vi "Compile Asynchronous Execution Units.vi"(0 "Device Ref in":T2=18446744073709551615 format="%.0x", 1 "Asynchronous Execution Units":T3[](array[typedef]) {"Outgoing Channels" format="%.0x"; "Incoming Channels" format="%.0x"}, 3 "error in":errorcluster) -> (7 "Device Ref out":T2=18446744073709551615 format="%.0x", 8 "Compiled Asynchronous Execution Units":T1[](array[typedef]), 10 "error out":errorcluster)   [LabVIEW 2020, in "Communication Bus Template System Explorer.lvlib" / "Implementation.lvlib"]
uses:
  Implementation.lvlib
  <vilib>/NI VeriStand/Custom Device API/Custom Device Item Ref.ctl
  <vilib>/NI VeriStand/Custom Device API/Custom Device API.lvlib
  <vilib>/NI/NIVS Inline Async API/_Data Access System Explorer/Data Access System Explorer.lvlib
  Engine/Interfaces/Execution Unit/Execution Unit.lvclass
  Engine/Custom Device/Asynchronous Execution Unit Compiled Information.ctl
  Engine/Custom Device/Custom Device.lvlib
  Engine/Interfaces/Controls/Execution Unit Information.ctl
  Engine/Interfaces/Interfaces.lvlib
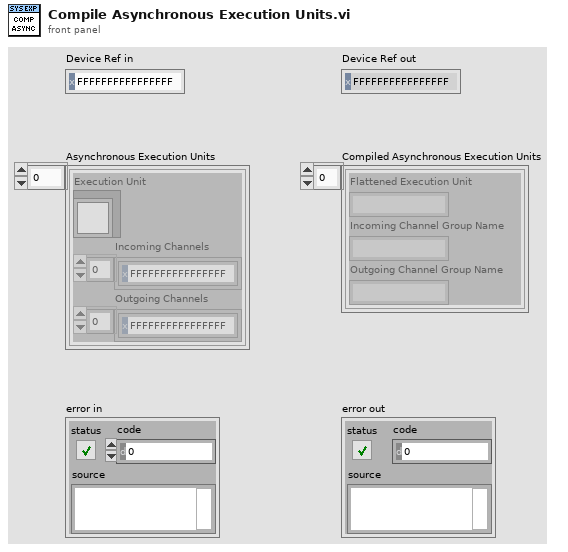
[diagram p1: front panel]
types:
  T1 = typedef "Communication Bus Template Engine.lvlib/Custom Device.lvlib/Asynchronous Execution Unit Compiled Information.ctl" = cluster{"Flattened Execution Unit":string, "Incoming Channel Group Name":string, "Outgoing Channel Group Name":string}
  T2 = typedef "Custom Device API.lvlib/Custom Device Item Ref.ctl" = u64
  T3 = typedef "Communication Bus Template Engine.lvlib/Interfaces.lvlib/Execution Unit Information.ctl" = cluster{"Execution Unit":refnum<class "Execution Unit.lvclass">, "Incoming Channels":T2[], "Outgoing Channels":T2[]}
  T4 = enum16{"Output/Write", "Input/Read", "Input/ReadWrite"}
  T5 = cluster{"Name":string, "Type":enum16{"Output/Write", "Input/Read", "Input/ReadWrite"}, "VS Refs":T2[]}
  T6 = cluster{"Name":string, "Type":enum16{"Output/Write", "Input/Read", "Input/ReadWrite"}, "VS Refs":T2[]}[]
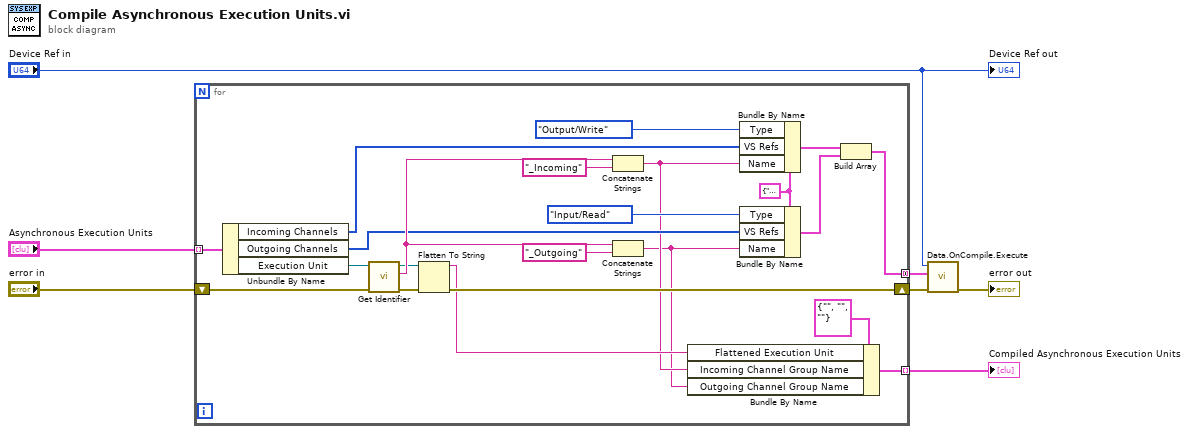
[diagram p0: block diagram]
diagram:
  n1 = for {
    tunnel: "Asynchronous Execution Units" -> [w28] mode=indexing
    tunnel: [w19] -> w6 mode=concatenating
    shift-right: [w18] -> w2
    shift-left: "error in" -> [w17]
    tunnel: [w11] -> w1 mode=indexing
    w10 = T5 {"Name"="", "Type"=enum."Output/Write", "VS Refs"=[]} ("Group")
    n2 = Unbundle By Name(w28) -> ("Incoming Channels"=w29:T2[], "Outgoing Channels"=w22:T2[], "Execution Unit"=w15:refnum<class "Execution Unit.lvclass">)
    n3 = call-dynamic "Get Identifier.vi"("error in (no error)"=w17, "Execution Unit in"=w15) -> ("error out"=w16:errorcluster, "Identifier"=w26:string, "Execution Unit out"=w14:refnum<class "Execution Unit.lvclass">)  [unwired: 7 in]
    n4 = Flatten To String(anything=w14, error in (no error)=w16) -> (data string=w12:string, error out=w18:errorcluster)  [unwired: 2 in, 1 out]
    n5 = Concatenate Strings(w26, "_Incoming" ("string")) -> (w9:string)
    n6 = Concatenate Strings(w26, "_Outgoing" ("string")) -> (w8:string)
    n7 = Bundle By Name(cluster=T1 {"Flattened Execution Unit"="", "Incoming Channel Group Name"="", "Outgoing Channel Group Name"=""} ("Asynchronous Execution Unit Compiled Information"), "Flattened Execution Unit"=w12, "Incoming Channel Group Name"=w9, "Outgoing Channel Group Name"=w8) -> (w11:T1)
    n8 = Bundle By Name(cluster=w10, "Type"=T4."Output/Write", "VS Refs"=w29, "Name"=w9) -> (w21:T5)
    n9 = Bundle By Name(cluster=w10, "Type"=T4."Input/Read", "VS Refs"=w22, "Name"=w8) -> (w20:T5)
    n10 = Build Array(w21, w20) -> (w19:T6)
  }
  "Compiled Asynchronous Execution Units" <- w1
  n11 = call <vilib>:"Data.OnCompile.Execute.vi"("error in"=w2, "VS Ref Groups"=w6, "Custom Device Ref"="Device Ref in") -> ("error out"=→"error out":errorcluster)  [unwired: 7 in, 1 out]
  "Device Ref out" <- "Device Ref in"
